vi "Coloring Doppler Demo.vi"() -> ()   [LabVIEW 2012]
uses:
  LabVIEW/user.lib/SpectralRadar.llb/Colorscheme Selection.ctl
  LabVIEW/user.lib/SpectralRadar.llb/Device Camera Preset Selection.ctl
  LabVIEW/user.lib/SpectralRadar.llb/Processing Parameter Int Selection.ctl
  LabVIEW/user.lib/SpectralRadar.llb/Coloring Byteorder.ctl
  LabVIEW/user.lib/SpectralRadar.llb/Doppler Property Int.ctl
  LabVIEW/user.lib/SpectralRadar.llb/Colored Data Export Format Selection.ctl
  LabVIEW/user.lib/SpectralRadar.llb/set Doppler Amplitude Output.vi
  LabVIEW/user.lib/SpectralRadar.llb/set Doppler Phase Output.vi
  LabVIEW/user.lib/SpectralRadar.llb/set Complex Scan Output.vi
  LabVIEW/user.lib/SpectralRadar.llb/OCT Device.lvclass
  LabVIEW/user.lib/SpectralRadar.llb/Probe.lvclass
  LabVIEW/user.lib/SpectralRadar.llb/Processing.lvclass
  LabVIEW/user.lib/SpectralRadar.llb/Raw Data.lvclass
  LabVIEW/user.lib/SpectralRadar.llb/Scan Pattern.lvclass
  LabVIEW/user.lib/SpectralRadar.llb/Coloring.lvclass
  LabVIEW/user.lib/SpectralRadar.llb/Colored Data.lvclass
  LabVIEW/user.lib/SpectralRadar.llb/LabVIEW Helper.lvlib
  LabVIEW/user.lib/SpectralRadar.llb/Complex Data.lvclass
  LabVIEW/user.lib/SpectralRadar.llb/Doppler Processing.lvclass
  LabVIEW/user.lib/SpectralRadar.llb/Data.lvclass
panel:
  in  "Averaging Z":i32=1
  in  "Averaging X":i32=2 min=2 max=20 step=1
  in  "Min Signal [dB]":sgl(slide)=1.4419259 min=-20 max=120 scale=-20.0..120.0
  in  "Doppler Boundaries":cluster{sgl, sgl}(slide)={1.4419259, -0.7006223} scale=-3.1415..3.1415
  in  "Save Button":bool
  in  "File Name":path
  in  "Display On/Off":bool=TRUE
  in  "Range":dbl=1.0
  in  "Color Table Selection":T1
  out "Averaged Frame Rate":dbl=6.134969234466553 format="%#_3g"
  out "Current Frame Rate":dbl=6.134969234466553 format="%#_3g"
  in  "Boundries":cluster{sgl, sgl}(slide)={76.65738, 42.00557} scale=-20.0..120.0
  out "Image":T2(plugin-control)
  in  "stop":bool
  in  "AScans":i32=1024
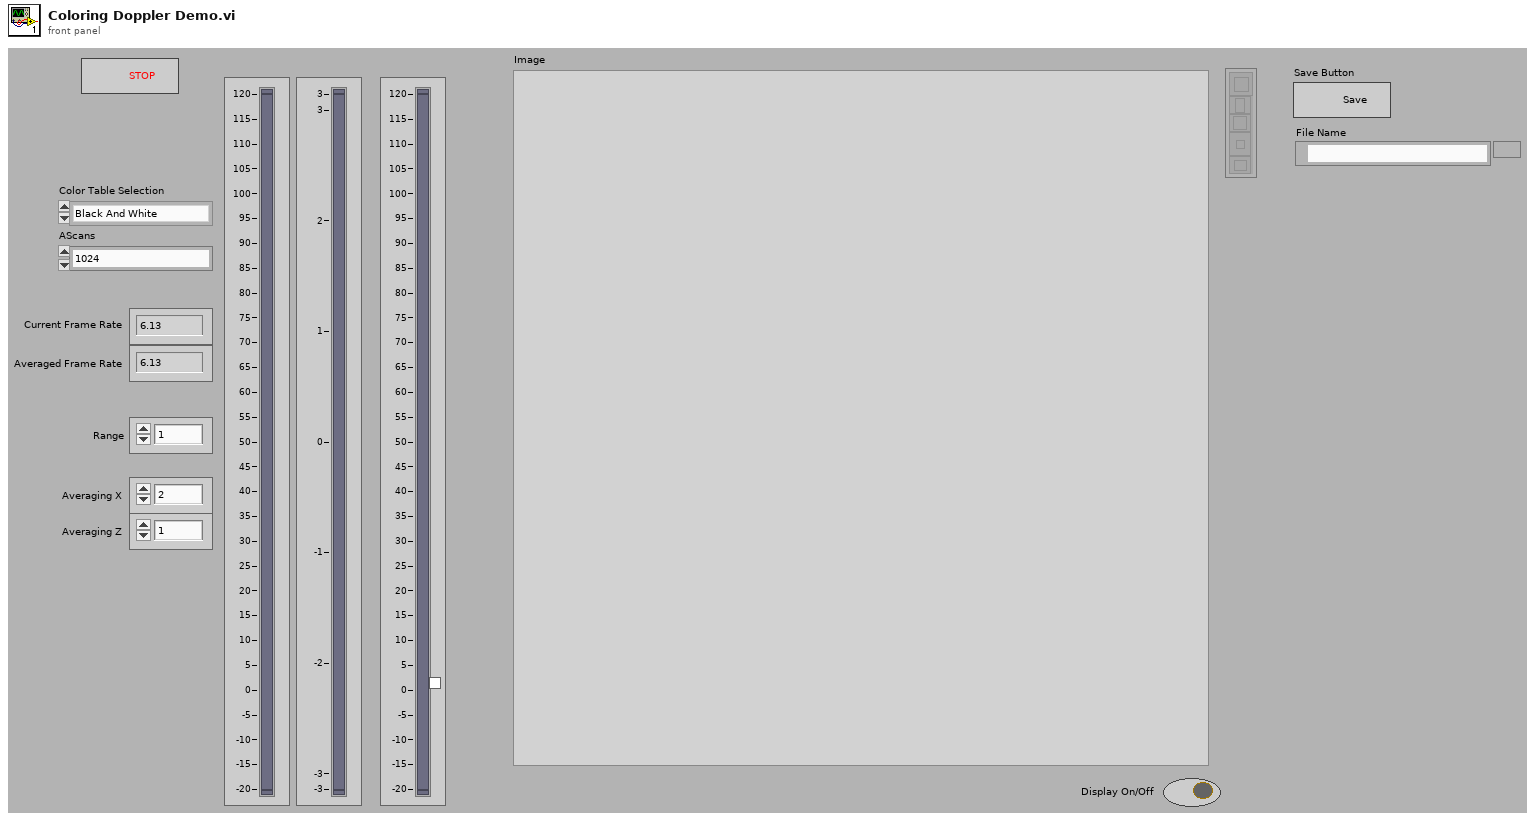
[diagram p1: front panel]
types:
  T1 = typedef "Coloring.lvclass/Colorscheme Selection.ctl" = enum16{"Black And White", "Inverted Black And White", "Color", "Black and Orange", "Black and Red", "Doppler Phase Coloring"}
  T2 = typedef "IMAQ Image.ctl" = refnum<image>
  T3 = typedef "Coloring.lvclass/Coloring Byteorder.ctl" = enum16{"RGBA32", "BGRA32", "ARGB32", ""}
  T4 = typedef "Processing.lvclass/Processing Parameter Int Selection.ctl" = enum32{"Spectrum Averaging", "A-Scan Averaging", "B-Scan Averaging", "Zero Padding", "Number of Threads", "Fourier Averaging"}
  T5 = typedef "OCT Device.lvclass/Device Camera Preset Selection.ctl" = enum16{"Default", "Preset 1", "Preset 2", "Preset 3"}
  T6 = typedef "Image Type" = u32
  T7 = enum16{"Asynchronous Continuous", "Asynchronous Finite", "Synchronous"}
  T8 = typedef "Doppler Processing.lvclass/Doppler Property Int.ctl" = enum16{"Doppler Averaging 1", "Doppler Averaging 2"}
  T9 = typedef "Colored Data.lvclass/Colored Data Export Format Selection.ctl" = enum16{"SRM (Spectral Radar Metafile)", "RAW", "BMP", "PNG", "JPG", "PDF", "TIFF"}
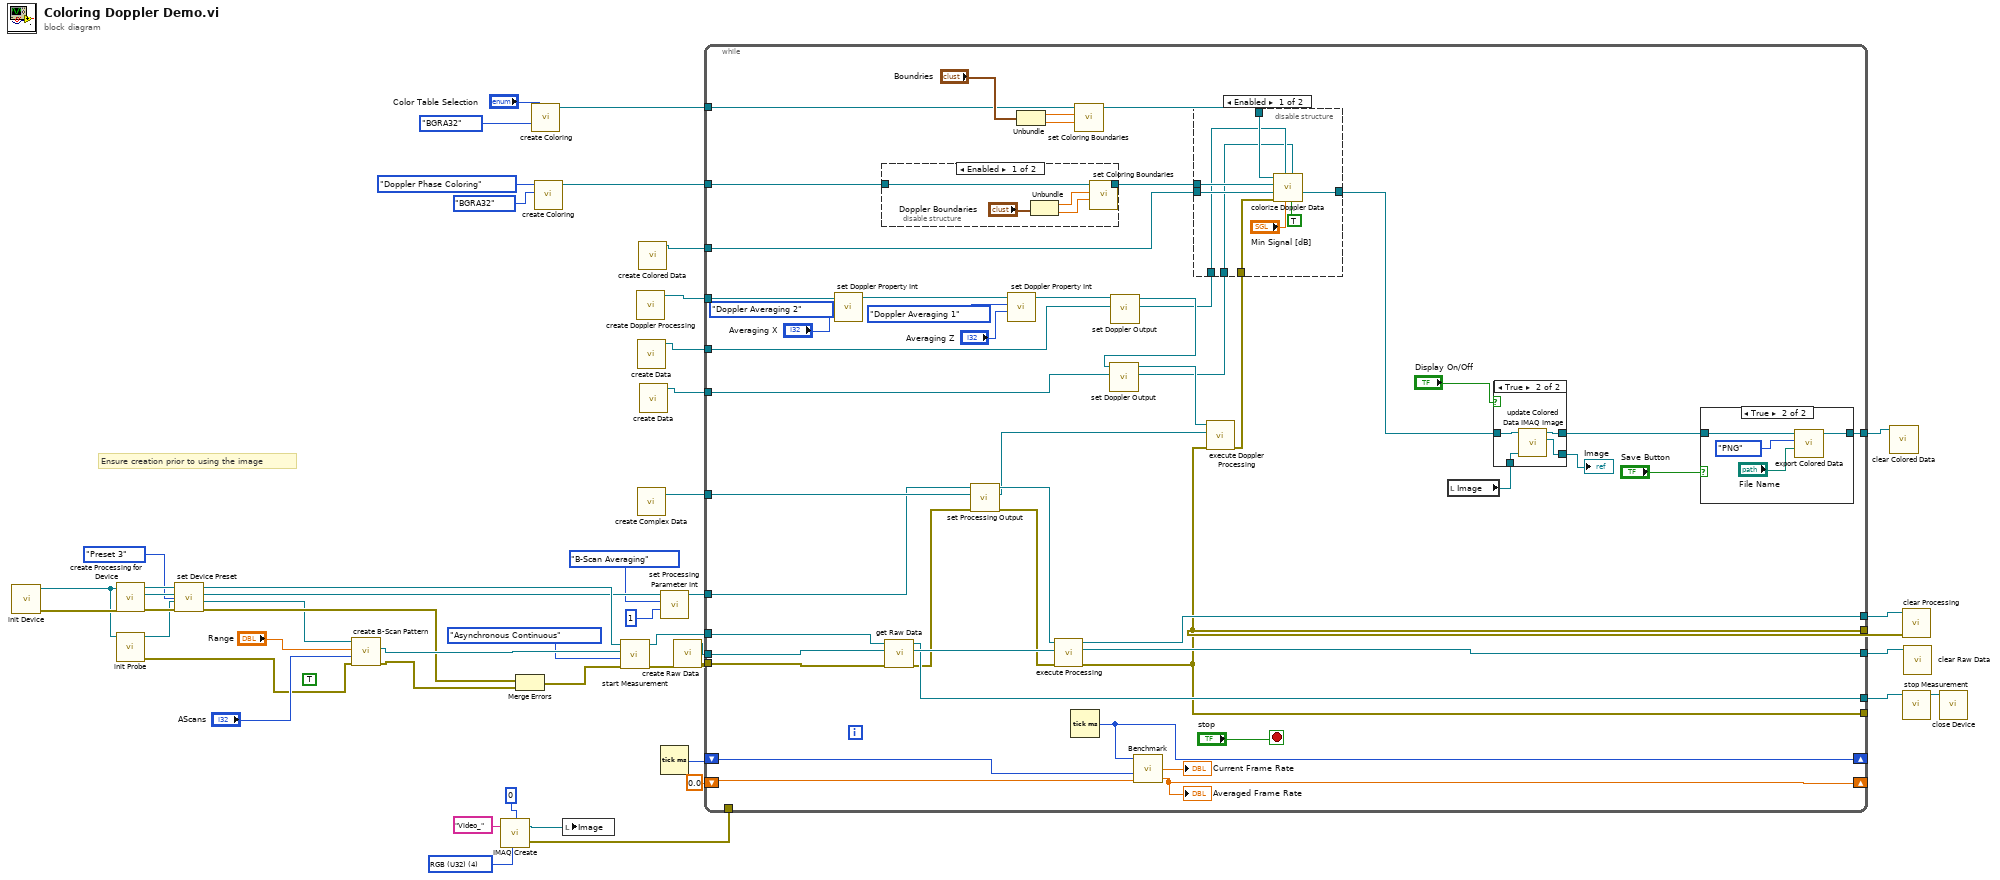
[diagram p0: block diagram]
diagram:
  (unwired) TRUE
  w29 = T6 4 items=["Grayscale (U8)", "Grayscale (I16)", "Grayscale (SGL)", "Complex (CSG)", "RGB (U32)", "HSL (U32)", "RGB (U64)", "Grayscale (U16)"] ("Image Type")
  # "Ensure creation prior to using the image"
  n1 = call "init Device.vi"() -> ("error out"=w48:errorcluster, "OCTDevice"=w18:refnum<class "OCT Device.lvclass">)  [unwired: 6 in]
  n2 = call "create Processing for Device.vi"("error in (no error)"=w48, "OCTDevice"=w18) -> ("error out"=w42:errorcluster, "Processing"=w22:refnum<class "Processing.lvclass">, "OCTDevice"=w23:refnum<class "OCT Device.lvclass">)  [unwired: 3 in]
  n3 = call "init Probe.vi"("OCT Device"=w18) -> ("error out"=w31:errorcluster, "GalvoControl"=w19:refnum<class "Probe.lvclass">)  [unwired: 5 in]
  n4 = call "set Device Preset.vi"("Numeric"=Device_Camera_Preset_Selection."Preset 3" ("Device Camera Preset Selection"), "Probe"=w19, "Processing"=w22, "OCTDevice"=w23) -> ("Probe 2"=w17:refnum<class "Probe.lvclass">, "Processing"=w14:refnum<class "Processing.lvclass">, "OCTDevice out"=w21:refnum<class "OCT Device.lvclass">)  [unwired: 2 in, 1 out]
  n5 = call "create B-Scan Pattern.vi"("error in (no error)"=w31, "AScans"="AScans", "Range"="Range", "Probe"=w17) -> ("error out"=w44:errorcluster, "Scan Pattern"=w46:refnum<class "Scan Pattern.lvclass">)  [unwired: 2 in, 1 out]
  n6 = call "IMAQ Create"("Border Size"=0, "Image Name"="Video_", "Image Type"=w29) -> ("New Image"=w27:T2, "error out"=w4:errorcluster)  [unwired: 2 in]
  n7 = Merge Errors(w42, w44) -> (w43:errorcluster)
  n8 = call "create Coloring.vi"("Color Byte Order"=Coloring_Byteorder."BGRA32", "Color Table Selection"="Color Table Selection") -> ("Coloring"=w26:refnum<class "Coloring.lvclass">)  [unwired: 4 in, 1 out]
  n9 = call "create Coloring.vi"("Color Byte Order"=Coloring_Byteorder."BGRA32", "Color Table Selection"=Colorscheme_Selection."Doppler Phase Coloring") -> ("Coloring"=w8:refnum<class "Coloring.lvclass">)  [unwired: 4 in, 1 out]
  n10 = local write "Image"(w27) -> ()
  n11 = call "start Measurement.vi"("error in (no error)"=w43, "Acquisition Type"=T7."Asynchronous Continuous", "Scan Pattern"=w46, "OCTDevice"=w21) -> ("error out"=w40:errorcluster, "OCTDevice"=w33:refnum<class "OCT Device.lvclass">)  [unwired: 1 in, 1 out]
  n12 = call "create Doppler Processing.vi"() -> ("Doppler Processing"=w6:refnum<class "Doppler Processing.lvclass">)  [unwired: 6 in, 1 out]
  n13 = call "create Data.vi"() -> ("Data"=w2:refnum<class "Data.lvclass">)  [unwired: 6 in, 1 out]
  n14 = call "create Complex Data.vi"() -> ("Complex Data"=w7:refnum<class "Complex Data.lvclass">)  [unwired: 2 in, 1 out]
  n15 = call "create Colored Data.vi"() -> ("Colored Data"=w3:refnum<class "Colored Data.lvclass">)  [unwired: 6 in, 1 out]
  n16 = call "create Data.vi"() -> ("Data"=w1:refnum<class "Data.lvclass">)  [unwired: 6 in, 1 out]
  n17 = call "set Processing Parameter Int.vi"("Value"=1, "Processing Paramter Int Selection"=Processing_Parameter_Int_Selection."B-Scan Averaging", "Processing in"=w14) -> ("Processing out"=w13:refnum<class "Processing.lvclass">)  [unwired: 3 in, 1 out]
  n18 = Tick Count (ms)() -> (millisecond timer value=w25:u32)
  n19 = call "create Raw Data.vi"("error in (no error)"=w40) -> ("error out"=w39:errorcluster, "Raw Data"=w41:refnum<class "Raw Data.lvclass">)  [unwired: 5 in]
  n20 = while {
    tunnel: w41 -> [w96]
    tunnel: w33 -> [w97]
    tunnel: w39 -> [w95]
    tunnel: w13 -> [w72]
    tunnel: [w92] -> w38
    tunnel: [w91] -> w37
    tunnel: [w90] -> w35
    tunnel: [w66] -> w36
    tunnel: [w66] -> _
    tunnel: w26 -> [w65]
    shift-right: [w82] -> _
    shift-left: w25 -> [w84]
    shift-right: [w81] -> _
    shift-left: sgl 0.0 ("AverageFrameRate") -> [w80]
    tunnel: [w76] -> w10
    tunnel: w8 -> [w74]
    tunnel: w7 -> [w73]
    tunnel: w6 -> [w53]
    tunnel: w2 -> [w71]
    tunnel: w1 -> [w69]
    tunnel: w4 -> [_]
    tunnel: w3 -> [w56]
    stop <- "stop" stop-if-true
    n21 = call "set Doppler Property Int.vi"("Value"="Averaging X", "Doppler Property"=Doppler_Property_Int."Doppler Averaging 2", "DopplerProcessing in"=w53) -> ("DopplerProcessing out"=w52:refnum<class "Doppler Processing.lvclass">)  [unwired: 3 in, 1 out]
    n22 = disable-structure shown="Enabled" {
      disable-tunnel: w74 -> [w112 w113]
      disable-tunnel: [w108 w113] -> w61
      frame Enabled {
        n23 = Unbundle("Doppler Boundaries") -> (w110:sgl, w109:sgl)
        n24 = call "set Coloring Boundaries.vi"("Danymic Range High [dB]"=w109, "Dynamic Range Low [dB]"=w110, "Coloring in"=w112) -> ("Coloring out"=w108:refnum<class "Coloring.lvclass">)  [unwired: 3 in, 1 out]
      }
      frame Disabled {
      }
    }
    n25 = call "get Raw Data.vi"("error in (no error)"=w95, "RawData in"=w96, "OCTDevice in"=w97) -> ("error out"=w89:errorcluster, "RawData out"=w93:refnum<class "Raw Data.lvclass">, "OCTDevice out"=w90:refnum<class "OCT Device.lvclass">)  [unwired: 2 in]
    n26 = call-poly "set Processing Output.vi"("error in (no error)"=w89, "Complex Data in"=w73, "Processing"=w72) -> ("error out"=w87:errorcluster, "Complex Data out"=w67:refnum<class "Complex Data.lvclass">, "Processing"=w94:refnum<class "Processing.lvclass">)  [unwired: 2 in]
    n27 = call "set Doppler Property Int.vi"("Value"="Averaging Z", "Doppler Property"=Doppler_Property_Int."Doppler Averaging 1", "DopplerProcessing in"=w52) -> ("DopplerProcessing out"=w55:refnum<class "Doppler Processing.lvclass">)  [unwired: 3 in, 1 out]
    n28 = Unbundle("Boundries") -> (w64:sgl, w63:sgl)
    n29 = call "execute Processing.vi"("error in (no error)"=w87, "Raw Data"=w93, "Processing"=w94) -> ("error out"=w66:errorcluster, "Raw Data"=w92:refnum<class "Raw Data.lvclass">, "Processing"=w91:refnum<class "Processing.lvclass">)  [unwired: 2 in]
    n30 = Tick Count (ms)() -> (millisecond timer value=w82:u32)
    n31 = call "set Coloring Boundaries.vi"("Danymic Range High [dB]"=w63, "Dynamic Range Low [dB]"=w64, "Coloring in"=w65) -> ("Coloring out"=w62:refnum<class "Coloring.lvclass">)  [unwired: 3 in, 1 out]
    n32 = call-poly "set Doppler Output.vi"("Data in"=w71, "DopplerProcessing in"=w55) -> ("Data out"=w60:refnum<class "Data.lvclass">, "DopplerProcessing out"=w70:refnum<class "Doppler Processing.lvclass">)  [unwired: 3 in, 1 out]
    n33 = call-poly "set Doppler Output.vi"("Data in"=w69, "DopplerProcessing in"=w70) -> ("Data out"=w59:refnum<class "Data.lvclass">, "DopplerProcessing out"=w68:refnum<class "Doppler Processing.lvclass">)  [unwired: 3 in, 1 out]
    n34 = call "Benchmark.vi"("Last Frame Rate"=w80, "TimeStart"=w84, "TimeFinish"=w82) -> ("AverageFrameRate"=w81:sgl, "FrameRate"=→"Current Frame Rate":sgl)  [unwired: 1 in, 1 out]
    "Averaged Frame Rate" <- w81
    n35 = call "execute Doppler Processing.vi"("error in (no error)"=w66, "Complex Data in"=w67, "DopplerProcessing in"=w68) -> ("error out"=w58:errorcluster)  [unwired: 2 in, 2 out]
    n36 = disable-structure shown="Enabled" {
      disable-tunnel: w62 -> [w106 _]
      disable-tunnel: w61 -> [w105 _]
      disable-tunnel: w56 -> [w104 w107]
      disable-tunnel: w60 -> [w103 _]
      disable-tunnel: w59 -> [w102 _]
      disable-tunnel: w58 -> [w101 _]
      disable-tunnel: [w100 w107] -> w57
      frame Enabled {
        n37 = call "colorize Doppler Data.vi"("Transpose"=TRUE, "Phase Data"=w102, "Min Signal [dB]"="Min Signal [dB]", "Amplitude Data"=w103, "error in (no error)"=w101, "Colored Data"=w104, "Phase Coloring in"=w105, "Amplitude Coloring in"=w106) -> ("Colored Data out"=w100:refnum<class "Colored Data.lvclass">)  [unwired: 3 out]
      }
      frame Disabled {
      }
    }
    n38 = local read "Image"() -> (w86:T2)
    n39 = case shown="True" "Display On/Off" {
      tunnel: w86 -> [w120 w124]
      tunnel: [w119 w123] -> w77
      tunnel: [w120 w122] -> w78
      tunnel: w57 -> [w119 w121]
      frame False {
      }
      frame True {
        n40 = call "update Colored Data IMAQ Image.vi"("Image in"=w124, "Colored Data"=w121) -> ("Image out"=w122:T2, "Colored Data"=w123:refnum<class "Colored Data.lvclass">)  [unwired: 3 in, 1 out]
      }
    }
    "Image" <- w78
    n41 = case shown="True" "Save Button" {
      tunnel: w77 -> [w114 w115]
      tunnel: [w114 w118] -> w76
      frame False {
      }
      frame True {
        n42 = call "export Colored Data.vi"("File Name"="File Name", "Colored Data Export Format Selection"=Colored_Data_Export_Format_Selection."PNG", "Colored Data in"=w115) -> ("Colored Data out"=w118:refnum<class "Colored Data.lvclass">)  [unwired: 3 in, 1 out]
      }
    }
  }
  n43 = call "clear Colored Data.vi"("Colored Data"=w10) -> ()  [unwired: 6 in, 1 out]
  n44 = call "clear Processing.vi"("error in (no error)"=w36, "Processing"=w37) -> ()  [unwired: 5 in, 1 out]
  n45 = call "stop Measurement.vi"("OCTDevice"=w35) -> ("OCTDevice"=w34:refnum<class "OCT Device.lvclass">)  [unwired: 5 in, 1 out]
  n46 = call "clear Raw Data.vi"("Raw Data"=w38) -> ()  [unwired: 6 in, 1 out]
  n47 = call "close Device.vi"("OCTDevice"=w34) -> ()  [unwired: 6 in, 1 out]
